vi "PH_Names.Famous Instances.vi"() -> (6 "Sequencer":string, 7 "Timing":string, 9 "PHELIX Beamline Chief":string, 10 "Z6 Beamline Chief":string)   [LabVIEW 2014, in "PH_Common.lvlib"]
uses:
  PH_Common.lvlib
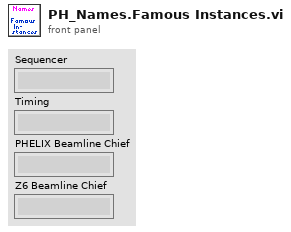
[diagram p1: front panel]
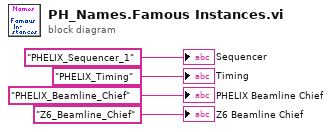
[diagram p0: block diagram]
diagram:
  "Timing" <- "PHELIX_Timing" ("Enabling Exp. 2.DIM Service Name")
  "Sequencer" <- "PHELIX_Sequencer_1" ("Enabling Exp. 1.DIM Service Name")
  "Z6 Beamline Chief" <- "Z6_Beamline_Chief" ("Enabling Exp. 2.DIM Service Name")
  "PHELIX Beamline Chief" <- "PHELIX_Beamline_Chief" ("Enabling Exp. 1.DIM Service Name")
